vi "例13.4 测量一段公式波形的频率.vi"() -> ()   [LabVIEW 2017]
uses:
  <vilib>/measure/matone.llb/Extract Single Tone Information 1 Chan.vi
  <vilib>/measure/NI_MAPro.lvlib
panel:
  in  "频率":dbl=1.0
  out "FFT频谱":cluster{"f0":dbl, "df":dbl, "magnitude":dbl[]}(graph)
  out "frequency":dbl caption="检测到的频率" format="%.2p"
  out "频率":dbl
  in  "formula":string="sin(2*w*t)+sin(3*w*t)" caption="公式"
  in  "采样信息":cluster{"Fs":dbl, "#s":dbl}={"Fs"=1000.0, "#s"=1000.0}
  out "f":dbl
  out "波形图":waveform(dbl)(graph)
  # "频率的测量结果"
  # "过零法"
  # "直接FFT法"
  # "提取单频信息"
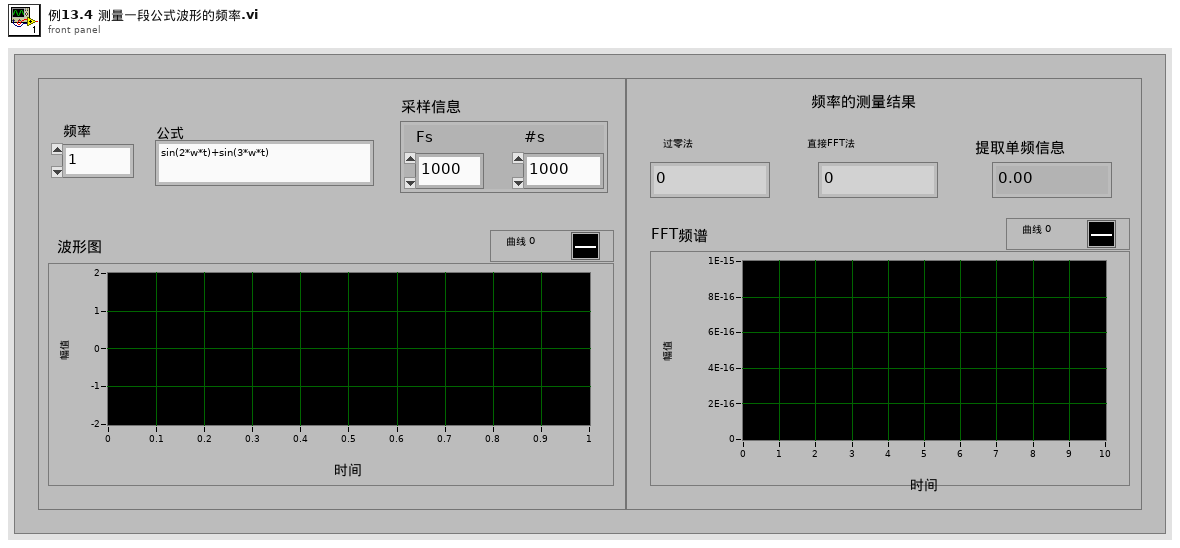
[diagram p1: front panel]
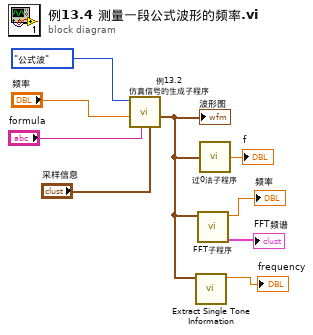
[diagram p0: block diagram]
diagram:
  n1 = call "例13.2 仿真信号的生成子程序.vi"("sampling info"="采样信息", "formula"="formula", "频率"="频率", "波形选择"=enum16{"正弦波", "三角波", "方波", "公式波"}."公式波") -> ("波形图"=w2:waveform(dbl))  [unwired: 7 in]
  "波形图" <- w2
  n2 = call-poly <vilib>:"Extract Single Tone Information.vi"("time signal in"=w2) -> ("detected frequency"=→"frequency":dbl)  [unwired: 5 in, 5 out]
  n3 = call "FFT子程序.vi"("time signal"=w2) -> ("FFT幅值"=→"FFT频谱":cluster{"f0":dbl, "df":dbl, "magnitude":dbl[]}, "频率"=→"频率":dbl)  [unwired: 3 in, 2 out]
  n4 = call "过0法子程序.vi"("波形"=w2) -> ("f"=→"f":dbl)
